vi "Module Type.vi"(11 "Sequence Submodule in":refnum<class "Sequence Submodule.lvclass">) -> (2 "Module Type":string)   [LabVIEW 2020, in "VolatusSeq.lvlib" / "Sequence Submodule.lvclass"]
uses:
  Sequence Submodule.lvclass
  Sequence Submodule.lvclass/Sequence Submodule.ctl
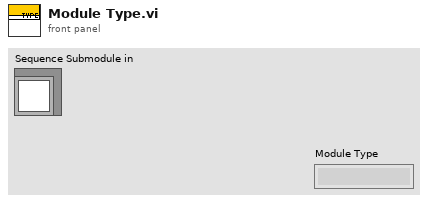
[diagram p1: front panel]
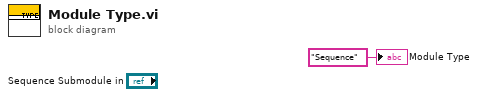
[diagram p0: block diagram]
diagram:
  "Module Type" <- "Sequence" ("Module Type")
